vi "test BroadcastRegistry2.vi"() -> ()   [LabVIEW 2014]
uses:
  user.lib/_NEVSTOP/Communicable State Machine(CSM)/_Support/Typedef/_CSM_Broadcast_Response_Message_info.ctl
  user.lib/_NEVSTOP/Communicable State Machine(CSM)/AdvanceAPI/CSM - Broadcast Message Type.ctl
  user.lib/_NEVSTOP/Communicable State Machine(CSM)/_Support/FGV-BroadcastRegistry/Operation-BroadcastRegistry.ctl
  user.lib/_NEVSTOP/Communicable State Machine(CSM)/Communicable State Machine.lvlib
panel:
  out "Cluster 10":cluster{"Registry":variant}
  out "Cluster 9":cluster{"Registry":variant}
  out "Cluster 8":cluster{"Registry":variant}
  out "Response Message Info":T1
  out "Cluster 7":cluster{"Registry":variant}
  out "Response Message Info":T1
  out "Cluster 6":cluster{"Registry":variant}
  out "Cluster 5":cluster{"Registry":variant}
  out "Cluster 4":cluster{"Registry":variant}
  out "Cluster 3":cluster{"Registry":variant}
  out "Response Message Info":T1
  out "Cluster 2":cluster{"Registry":variant}
  out "Response Message Info":T1
  out "Cluster":cluster{"Registry":variant}
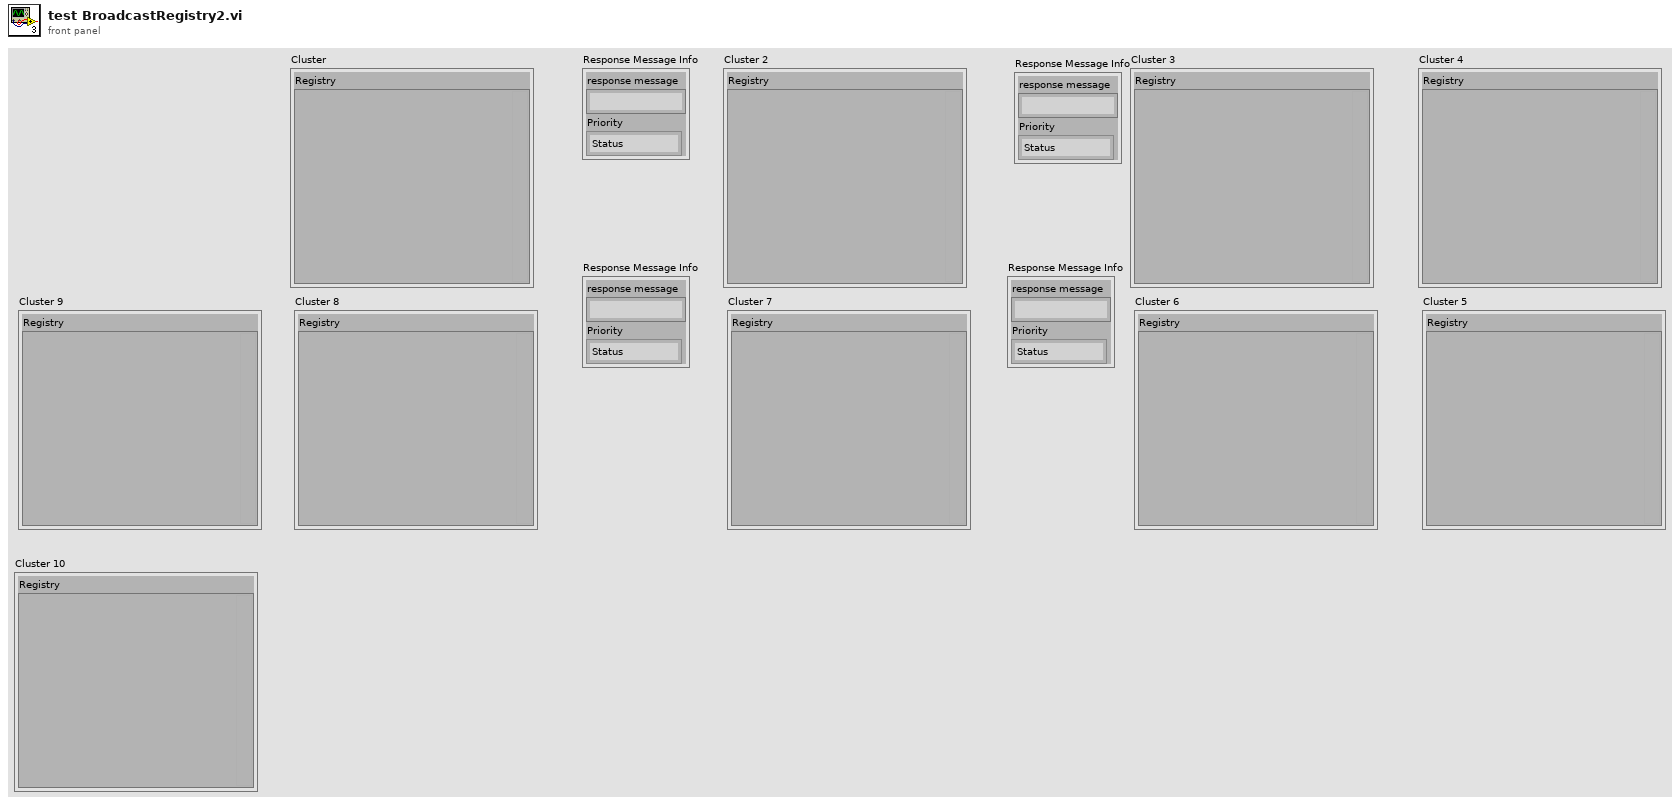
[diagram p1: front panel]
types:
  T1 = typedef "Communicable State Machine.lvlib/_CSM_Broadcast_Response_Message_info.ctl" = cluster{"response message":string, "Priority":T2}
  T2 = typedef "Communicable State Machine.lvlib/CSM - Broadcast Message Type.ctl" = enum16{"Status", "Interrupt(High)"}
  T3 = typedef "Communicable State Machine.lvlib/Operation-BroadcastRegistry.ctl" = enum16{"Delete Source Module", "Delete Target Module", "Remove Module", "Register", "Unregister", "Check"}
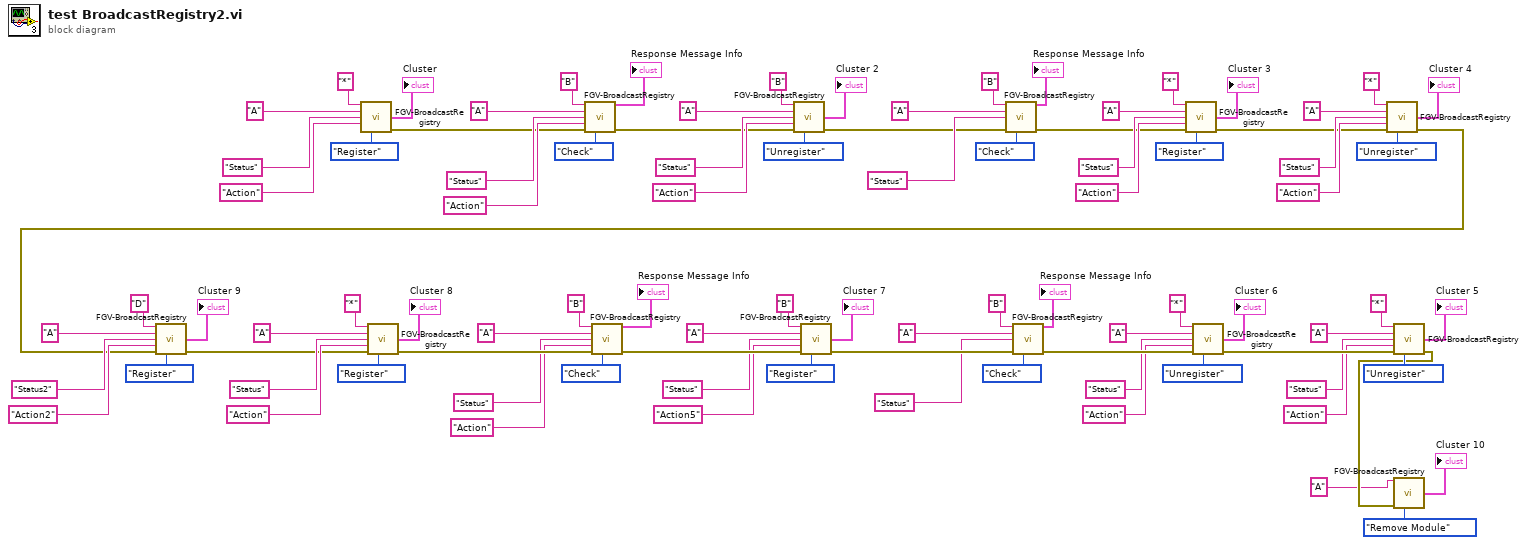
[diagram p0: block diagram]
diagram:
  n1 = call "FGV-BroadcastRegistry.vi"("Source"="*", "Target"="A" ("Dest"), "Message"="Status", "Response Message In"="Action", "Operation"=Operation-BroadcastRegistry."Register") -> ("Cluster"=→"Cluster":cluster{"Registry":variant}, "Error out"=w81:errorcluster)  [unwired: 8 in, 1 out]
  n2 = call "FGV-BroadcastRegistry.vi"("Source"="B", "Target"="A" ("Dest"), "Message"="Status", "Response Message In"="Action", "Error in"=w81, "Operation"=Operation-BroadcastRegistry."Check") -> ("Response Message Info"=→"Response Message Info":T1, "Error out"=w73:errorcluster)  [unwired: 7 in, 1 out]
  n3 = call "FGV-BroadcastRegistry.vi"("Source"="B", "Target"="A" ("Dest"), "Message"="Status", "Response Message In"="Action", "Error in"=w73, "Operation"=Operation-BroadcastRegistry."Unregister") -> ("Cluster"=→"Cluster 2":cluster{"Registry":variant}, "Error out"=w67:errorcluster)  [unwired: 7 in, 1 out]
  n4 = call "FGV-BroadcastRegistry.vi"("Source"="B", "Target"="A" ("Dest"), "Message"="Status", "Error in"=w67, "Operation"=Operation-BroadcastRegistry."Check") -> ("Response Message Info"=→"Response Message Info":T1, "Error out"=w60:errorcluster)  [unwired: 8 in, 1 out]
  n5 = call "FGV-BroadcastRegistry.vi"("Source"="*", "Target"="A" ("Dest"), "Message"="Status", "Response Message In"="Action", "Error in"=w60, "Operation"=Operation-BroadcastRegistry."Register") -> ("Cluster"=→"Cluster 3":cluster{"Registry":variant}, "Error out"=w53:errorcluster)  [unwired: 7 in, 1 out]
  n6 = call "FGV-BroadcastRegistry.vi"("Source"="*", "Target"="A" ("Dest"), "Message"="Status", "Response Message In"="Action", "Error in"=w53, "Operation"=Operation-BroadcastRegistry."Unregister") -> ("Cluster"=→"Cluster 4":cluster{"Registry":variant}, "Error out"=w6:errorcluster)  [unwired: 7 in, 1 out]
  n7 = call "FGV-BroadcastRegistry.vi"("Source"="D", "Target"="A" ("Dest"), "Message"="Status2", "Response Message In"="Action2", "Error in"=w6, "Operation"=Operation-BroadcastRegistry."Register") -> ("Cluster"=→"Cluster 9":cluster{"Registry":variant}, "Error out"=w5:errorcluster)  [unwired: 7 in, 1 out]
  n8 = call "FGV-BroadcastRegistry.vi"("Source"="*", "Target"="A" ("Dest"), "Message"="Status", "Response Message In"="Action", "Error in"=w5, "Operation"=Operation-BroadcastRegistry."Register") -> ("Cluster"=→"Cluster 8":cluster{"Registry":variant}, "Error out"=w24:errorcluster)  [unwired: 7 in, 1 out]
  n9 = call "FGV-BroadcastRegistry.vi"("Source"="B", "Target"="A" ("Dest"), "Message"="Status", "Response Message In"="Action", "Error in"=w24, "Operation"=Operation-BroadcastRegistry."Check") -> ("Response Message Info"=→"Response Message Info":T1, "Error out"=w32:errorcluster)  [unwired: 7 in, 1 out]
  n10 = call "FGV-BroadcastRegistry.vi"("Source"="B", "Target"="A" ("Dest"), "Message"="Status", "Response Message In"="Action5", "Error in"=w32, "Operation"=Operation-BroadcastRegistry."Register") -> ("Cluster"=→"Cluster 7":cluster{"Registry":variant}, "Error out"=w38:errorcluster)  [unwired: 7 in, 1 out]
  n11 = call "FGV-BroadcastRegistry.vi"("Source"="B", "Target"="A" ("Dest"), "Message"="Status", "Error in"=w38, "Operation"=Operation-BroadcastRegistry."Check") -> ("Response Message Info"=→"Response Message Info":T1, "Error out"=w45:errorcluster)  [unwired: 8 in, 1 out]
  n12 = call "FGV-BroadcastRegistry.vi"("Source"="*", "Target"="A" ("Dest"), "Message"="Status", "Response Message In"="Action", "Error in"=w45, "Operation"=Operation-BroadcastRegistry."Unregister") -> ("Cluster"=→"Cluster 6":cluster{"Registry":variant}, "Error out"=w52:errorcluster)  [unwired: 7 in, 1 out]
  n13 = call "FGV-BroadcastRegistry.vi"("Source"="*", "Target"="A" ("Dest"), "Message"="Status", "Response Message In"="Action", "Error in"=w52, "Operation"=Operation-BroadcastRegistry."Unregister") -> ("Cluster"=→"Cluster 5":cluster{"Registry":variant}, "Error out"=w2:errorcluster)  [unwired: 7 in, 1 out]
  n14 = call "FGV-BroadcastRegistry.vi"("Source"="A" ("Dest"), "Error in"=w2, "Operation"=Operation-BroadcastRegistry."Remove Module") -> ("Cluster"=→"Cluster 10":cluster{"Registry":variant})  [unwired: 10 in, 2 out]
